vi "Scarta plot interpolazioni.vi"(10 "GRAFICO QH":cluster{"X":dbl[], "Y":dbl[]}[](array[cluster]), 11 "XYGraph in":refnum<vi>) -> ()   [LabVIEW 2019]
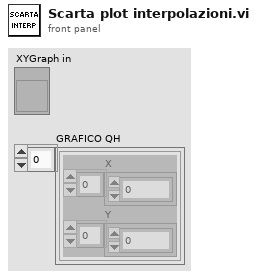
[diagram p1: front panel]
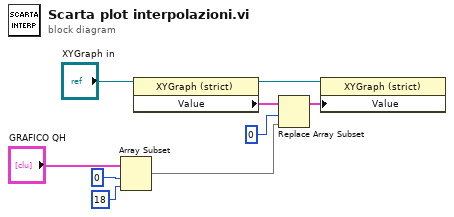
[diagram p0: block diagram]
diagram:
  n1 = Array Subset(array="GRAFICO QH", index=0, length=18) -> (w6:cluster{"X":dbl[], "Y":dbl[]}[])
  n2 = property class="XYGraph (strict)"(reference="XYGraph in") -> (reference out=w2:refnum<vi>, "Value"=w3:cluster{"X":dbl[], "Y":dbl[]}[])  [unwired: 1 in, 1 out]
  n3 = Replace Array Subset(array=w3, new element=w6, index=0) -> (w1:cluster{"X":dbl[], "Y":dbl[]}[])
  n4 = property class="XYGraph (strict)"(reference=w2, "Value"=w1) -> ()  [unwired: 1 in, 2 out]
